vi "Hide Panel.vi"(7 "Connection Name":string, 8 "error in (no error)":errorcluster, 11 "Module ID":i32=-1) -> (0 "error out":errorcluster)   [LabVIEW 2017, in "SSH.lvlib"]
doc: "Send the Hide Panel request to the Module's Main.vi.\n_____\nBased on Delacor QMH Project Template 4.2.1.64."
uses:
  SSH.lvlib
  Hide Panel Argument--cluster.ctl
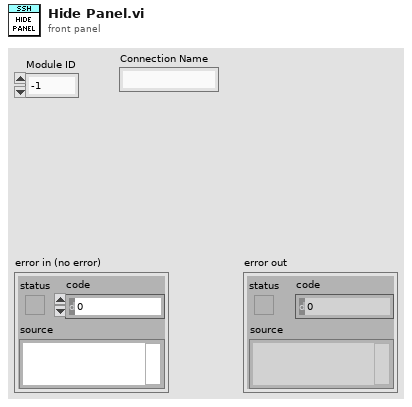
[diagram p1: front panel]
types:
  T1 = typedef "SSH.lvlib/Hide Panel Argument--cluster.ctl" = cluster{"Module ID":i32, "Hide Panel?":bool}
  T2 = typedef "SSH.lvlib/Request Events--cluster.ctl" = cluster{"Stop Module":refnum<user-event>, "Show Panel":refnum<user-event>, "Hide Panel":refnum<user-event>, "Show Diagram":refnum<user-event>, "Get Module Execution Status":refnum<user-event>, "Write Command":refnum<user-event>}
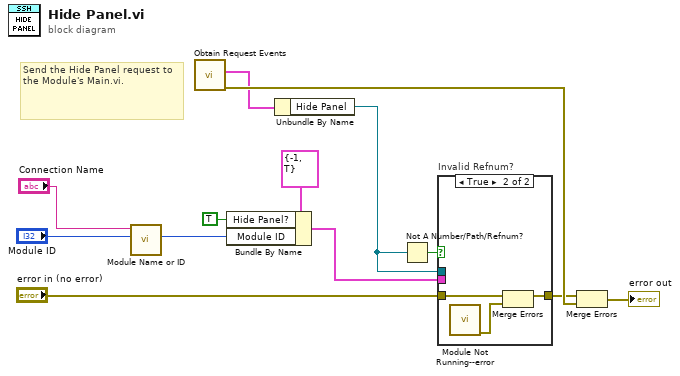
[diagram p0: block diagram]
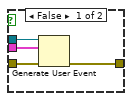
[diagram p2: hidden frame]
diagram:
  # "Send the Hide Panel request to the Module's Main.vi."
  n1 = call "Module Name or ID.vi"("Module ID in"="Module ID", "Connection Name"="Connection Name") -> ("Module ID out"=w2:i32)  [unwired: 9 in]
  n2 = call "Obtain Request Events.vi"() -> ("error out"=w12:errorcluster, "SSH Request Events"=w11:T2)  [unwired: 10 in]
  n3 = Bundle By Name(cluster=T1 {"Module ID"=-1, "Hide Panel?"=TRUE} ("Hide Panel Argument"), "Hide Panel?"=TRUE ("event data"), "Module ID"=w2) -> (w3:T1)
  n4 = Unbundle By Name(w11) -> ("Hide Panel"=w5:refnum<user-event>)
  n5 = Not A Number/Path/Refnum?(number/path/refnum=w5) -> (NaN/Path/Refnum?=w7:bool)
  n6 = case "Invalid Refnum?" shown="True" w7 {
    tunnel: "error in (no error)" -> [w17 w18]
    tunnel: [w16 w19] -> w6
    tunnel: w3 -> [w15 _]
    tunnel: w5 -> [w14 _]
    frame False {
      n7 = Generate User Event(user event=w14, event data cluster=w15, error in=w17) -> (error out=w16:errorcluster)  [unwired: 1 in, 1 out]
    }
    frame True {
      n8 = call "Module Not Running--error.vi"() -> ("error out"=w20:errorcluster)  [unwired: 11 in]
      n9 = Merge Errors(w18, w20) -> (w19:errorcluster)
    }
  }
  n10 = Merge Errors(w6, w12) -> (→"error out":errorcluster)
